vi "CavityFilter.vi"(7 "Reset":bool=TRUE, 8 "input valid":bool=TRUE, 9 "b":fxp<+/-,32,17>, 10 "a":fxp<+/-,32,4>, 11 "Value in":fxp<+/-,32,14>) -> (0 "output valid":bool, 3 "Value out":fxp<+/-,32,14>)   [LabVIEW 2018]
doc: "Caclulate\ny(n) = a * x(n-1) + b * ( x(n) - x(n-1) )"
uses:
  <vilib>/rvi/FXPMathLib/FxpConvert/subVIs/nifxpmath_Convert_SimConfig.ctl
  <vilib>/fxp/LVFixedPointQuantizationPolicyTypeDef.ctl
  <vilib>/fxp/LVFixedPointOverflowPolicyTypeDef.ctl
  <vilib>/rvi/FXPMathLib/FxpConvert/simVIs/DllFxpConvertTemp_sub.vi
  <vilib>/rvi/FXPMathLib/FxpAdd/XNode/nifxpmath_Add.xnode
  <vilib>/rvi/FXPMathLib/FxpConvert/XNode/nifxpmath_Convert.xnode
  <vilib>/rvi/FXPMathLib/FxpSub/XNode/nifxpmath_Sub.xnode
  <vilib>/rvi/FXPMathLib/FxpMul/XNode/nifxpmath_Multiplier.xnode
  <vilib>/rvi/FXPMathLib/sim/FxpSim.dll
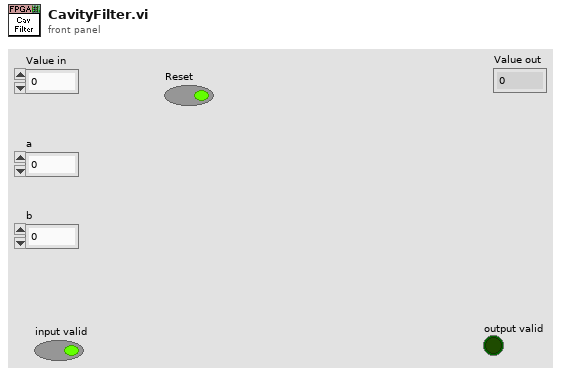
[diagram p1: front panel]
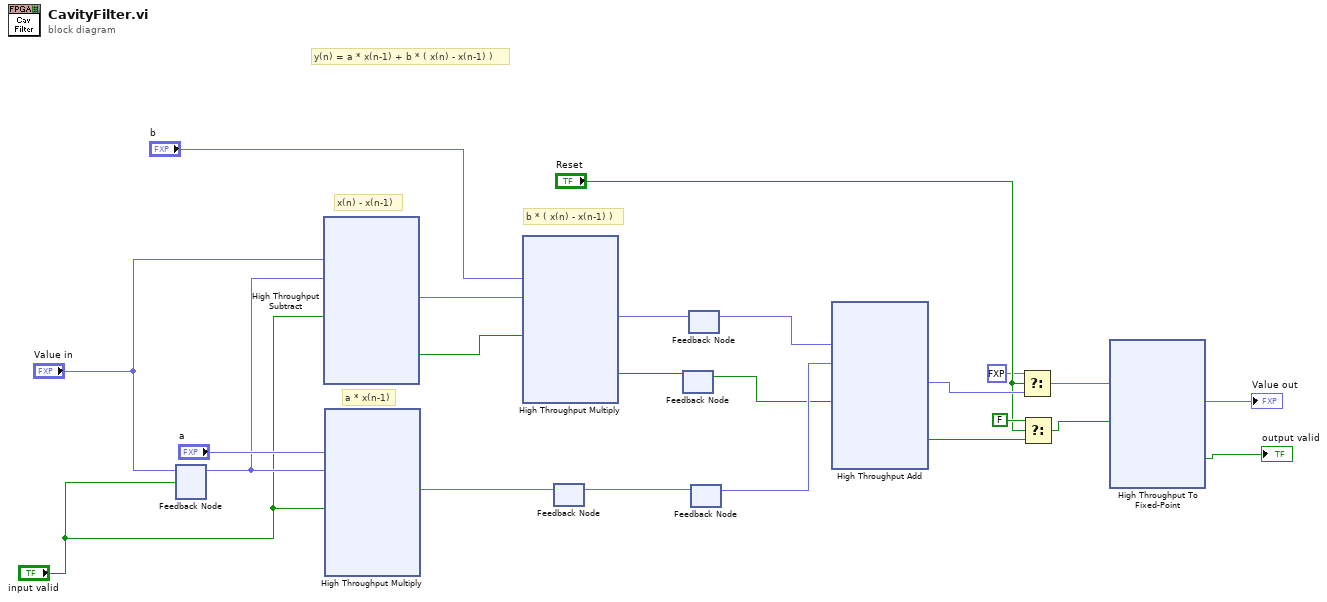
[diagram p0: block diagram]
diagram:
  # "b * ( x(n) - x(n-1) )"
  # "a * x(n-1)"
  # "x(n) - x(n-1)"
  # "y(n) = a * x(n-1) + b * ( x(n) - x(n-1) )"
  n1 = feedback-in #1("Value in", "input valid") -> ()
  n2 = feedback #1() -> (w16:fxp<+/-,32,14>)  [unwired: 1 in]
  n3 = xnode "High Throughput Subtract"("x"="Value in", "y"=w16, "input valid"="input valid") -> ("x-y"=w13:fxp<+/-,33,15>, "output valid"=w12:bool)  [unwired: 1 in, 1 out]
  n4 = xnode ("High Throughput Multiply")("x"="a", "y"=w16, "input valid"="input valid") -> ("x*y"=w6:fxp<+/-,48,18>)  [unwired: 1 in, 2 out]
  n5 = xnode ("High Throughput Multiply")("x"="b", "y"=w13, "input valid"=w12) -> ("x*y"=w23:fxp<+/-,48,32>, "output valid"=w10:bool)  [unwired: 1 in, 1 out]
  n6 = feedback #2() -> (w11:fxp<+/-,48,18>)  [unwired: 1 in]
  n7 = feedback-in #2(w6) -> ()
  n8 = feedback #3() -> (w7:bool)  [unwired: 1 in]
  n9 = feedback-in #3(w10) -> ()
  n10 = feedback #4() -> (w9:fxp<+/-,48,32>)  [unwired: 1 in]
  n11 = feedback-in #4(w23) -> ()
  n12 = feedback #5() -> (w8:fxp<+/-,48,18>)  [unwired: 1 in]
  n13 = feedback-in #5(w11) -> ()
  n14 = xnode ("High Throughput Add")("x"=w9, "y"=w8, "input valid"=w7) -> ("x+y"=w21:fxp<+/-,63,33>, "output valid"=w20:bool)  [unwired: 1 in, 1 out]
  n15 = Select(t=fxp<+/-,63,33> 0.0, s="Reset", f=w21) -> (s? t:f=w4:fxp<+/-,63,33>)
  n16 = Select(t=FALSE, s="Reset", f=w20) -> (s? t:f=w5:bool)
  n17 = xnode "High Throughput To Fixed-Point"("x"=w4, "input valid"=w5) -> ("y"=→"Value out":fxp<+/-,32,14>, "output valid"=→"output valid":bool)  [unwired: 1 in, 1 out]
